vi "API_DB.ExecuteSQlCommand.vi"(6 "Timeout (ms)":u32, 7 "Wait (F)":bool, 8 "error in (no error)":errorcluster, 10 "SQLCommand":string, 11 "Database in":refnum<class "Database.lvclass">) -> (0 "error out":errorcluster, 2 "Return Value":variant, 3 "Database out":refnum<class "Database.lvclass">)   [LabVIEW 2022 SP3, in "Database.lvclass"]
doc: "Developed by Kevin Thompson\nkevin@thompsonengineering.net\n\nCopyright 2018\nThompson Engineering, LLC"
uses:
  Database.lvclass
  DataTypes/AsynCmd_Temp01--enum.ctl
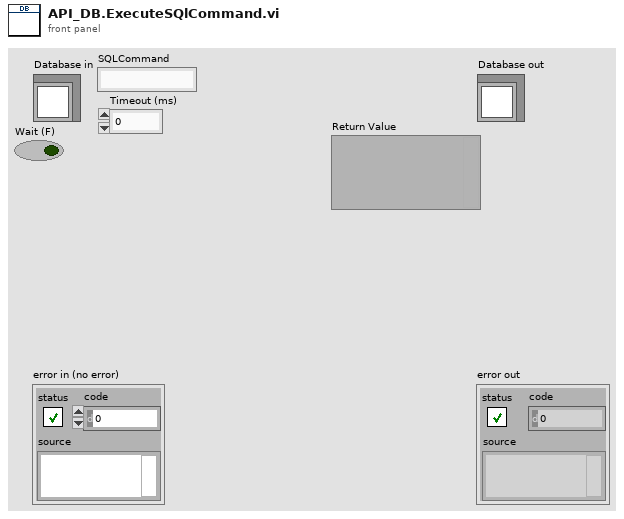
[diagram p1: front panel]
types:
  T1 = typedef "Database.lvclass/AsynCmd_Temp01--enum.ctl" = enum16{"DB.DeleteRecord", "DB.UpdateRecord", "DB.InsertRecord", "DB.SelectRecord", "DB.ExecuteSQLCommand", "DB.FindFirstSlot", "DB.GenericSQLQuery"}
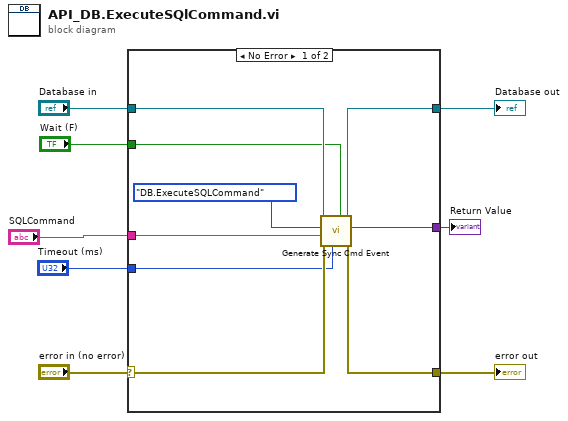
[diagram p0: block diagram]
diagram:
  n1 = case shown="No Error" "error in (no error)" {
    selector: "error in (no error)" -> [w15 w19]
    tunnel: [w14 w19] -> w7
    tunnel: [w16 w18] -> w5
    tunnel: "Database in" -> [w17 w18]
    tunnel: "SQLCommand" -> [w12 _]
    tunnel: "Wait (F)" -> [w11 _]
    tunnel: "Timeout (ms)" -> [w10 _]
    tunnel: [w9 _] -> w1
    frame No Error {
      n2 = call "Generate Sync Cmd Event.vi"("Wait (F)"=w11, "Timeout (ms)"=w10, "error in (no error)"=w15, "vData"=w12, "AsyncCmd"=AsynCmd_Temp01--enum."DB.ExecuteSQLCommand", "Database in"=w17) -> ("error out"=w14:errorcluster, "Return Value"=w9:variant, "Database out"=w16:refnum<class "Database.lvclass">)  [unwired: 3 in]
    }
    frame Error {
    }
  }
  "error out" <- w7
  "Database out" <- w5
  "Return Value" <- w1
